vi "ResMgr-Request PriorityQueue.vi"(6 "Timeout In ms (5000 ms)":i32=5000, 7 "WatchDogQ":refnum<queue>, 8 "Error In":errorcluster caption="error in (no error)") -> (0 "error out":errorcluster, 3 "Priority Queue":T1)   [LabVIEW 2017, in "Communicable State Machine.lvlib"]
uses:
  Communicable State Machine.lvlib
  Priority Queue/Priority Queue.ctl
  Typedef/_Cross CSM State Data.ctl
  Typedef/_CSM_MSG_TYPE.ctl
  Typedef/_Cross CSM State Response.ctl
  Typedef/_CSM_Response Source Message.ctl
  Priority Queue/def-Data(LowPRI-Q).ctl
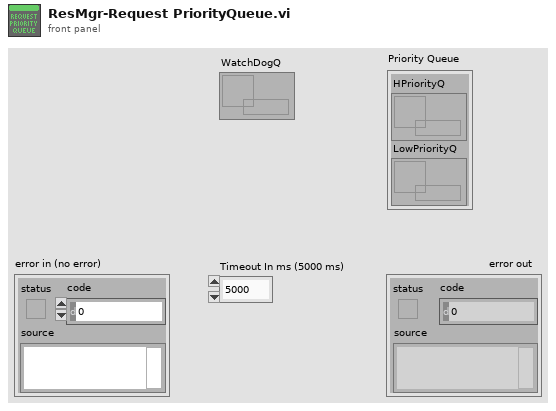
[diagram p1: front panel]
types:
  T1 = typedef "Communicable State Machine.lvlib/Priority Queue.ctl" = cluster{"HPriorityQ":refnum<queue>, "LowPriorityQ":refnum<queue>}
  T2 = cluster{"ResType":string, "RespQ":refnum<queue>, "Parameter":string, "WatchDogQ":refnum<queue>}
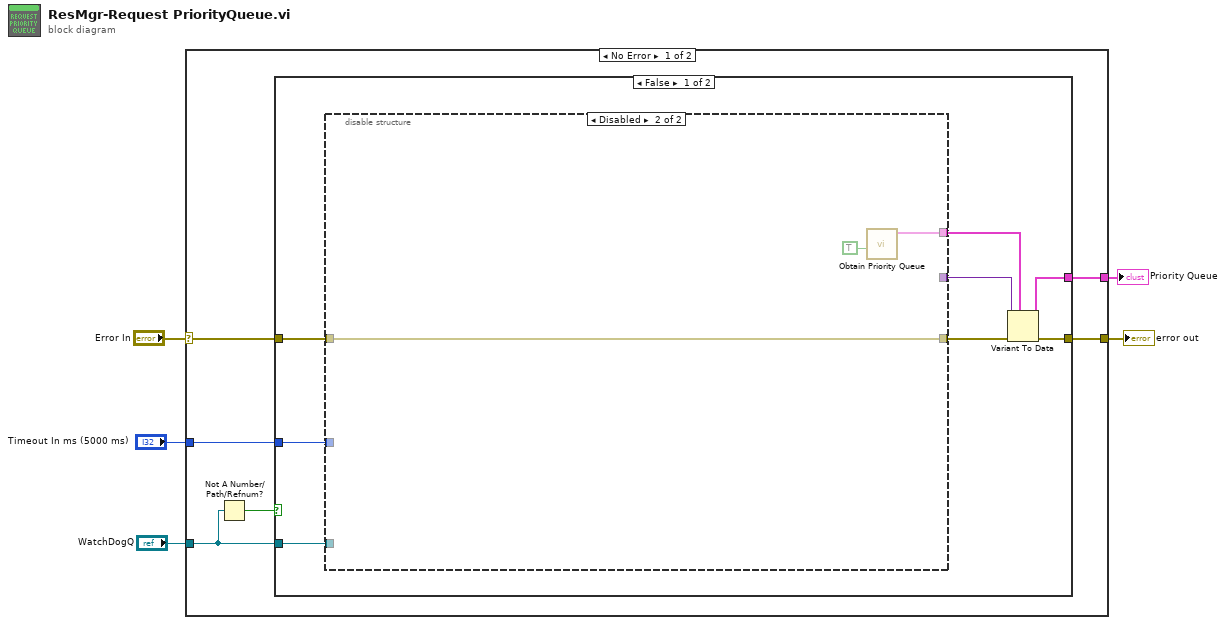
[diagram p0: block diagram]
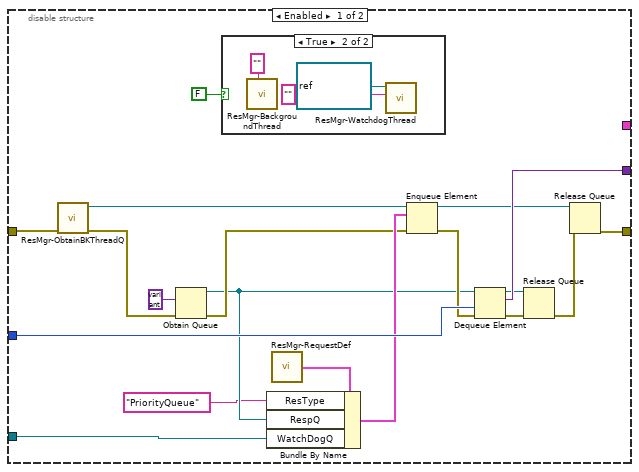
[diagram p2: hidden frame]
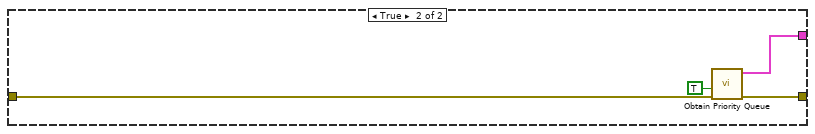
[diagram p4: hidden frame]
diagram:
  n1 = case shown="No Error" "Error In" {
    selector: "Error In" -> [w10 w49]
    tunnel: [w9 w49] -> w5
    tunnel: [w8 _] -> w1
    tunnel: "Timeout In ms (5000 ms)" -> [w11 _]
    tunnel: "WatchDogQ" -> [w7 _]
    frame No Error {
      n2 = Not A Number/Path/Refnum?(number/path/refnum=w7) -> (NaN/Path/Refnum?=w6:bool)
      n3 = case shown="False" w6 {
        tunnel: w11 -> [w18 _]
        tunnel: w10 -> [w17 w45]
        tunnel: w7 -> [w16 _]
        tunnel: [w15 w47] -> w9
        tunnel: [w12 w46] -> w8
        frame False {
          n4 = disable-structure shown="Disabled" {
            disable-tunnel: [w38 w44] -> w19
            disable-tunnel: w18 -> [w37 _]
            disable-tunnel: [w36 _] -> w14
            disable-tunnel: w17 -> [w23 w44]
            disable-tunnel: w16 -> [w22 _]
            disable-tunnel: [_ w42] -> w13
            frame Enabled {
              n5 = call "ResMgr-ObtainBKThreadQ.vi"("error in (no error)"=w23) -> ("error out"=w33:errorcluster, "ObtainBKThreadQ"=w34:refnum<queue>)  [unwired: 9 in]
              n6 = Obtain Queue(element data type=variant, error in (no error)=w33) -> (queue out=w24:refnum<queue>, error out=w32:errorcluster)  [unwired: 3 in, 1 out]
              n7 = case shown="True" FALSE {
                frame False {
                }
                frame True {
                  n8 = call "ResMgr-BackgroundThread.vi"("Name (Unnamed)"="" ("name (unnamed)")) -> ()  [unwired: 11 in]
                  n9 = call "ResMgr-WatchdogThread.vi"("From Who"="", "WatchDogQ"=refnum<queue> refnum) -> ()  [unwired: 10 in]
                }
              }
              n10 = call "ResMgr-RequestDef.vi"() -> ("ResMgr-RequestDef.ctl"=w20:T2)  [unwired: 2 in]
              n11 = Bundle By Name(cluster=w20, "ResType"="PriorityQueue", "RespQ"=w24, "WatchDogQ"=w22) -> (w35:T2)
              n12 = Enqueue Element(queue=w34, element=w35, error in (no error)=w32) -> (queue out=w28:refnum<queue>, error out=w31:errorcluster)  [unwired: 1 in, 1 out]
              n13 = Dequeue Element(queue=w24, timeout in ms (-1)=w37, error in (no error)=w31) -> (queue out=w29:refnum<queue>, element=w36:variant, error out=w30:errorcluster)  [unwired: 1 out]
              n14 = Release Queue(queue=w29, error in (no error)=w30) -> (error out=w27:errorcluster)  [unwired: 1 in, 2 out]
              n15 = Release Queue(queue=w28, error in (no error)=w27) -> (error out=w38:errorcluster)  [unwired: 1 in, 2 out]
            }
            frame Disabled {
              n16 = call "Obtain Priority Queue.vi"("Create If Not Found? (T)"=TRUE ("create if not found? (T)")) -> ("Priority Queue"=w42:T1)  [unwired: 8 in, 2 out]
            }
          }
          n17 = Variant To Data(error in=w19, type=w13, Variant=w14) -> (data=w12:T1, error out=w15:errorcluster)
        }
        frame True {
          n18 = call "Obtain Priority Queue.vi"("error in (no error)"=w45, "Create If Not Found? (T)"=TRUE ("create if not found? (T)")) -> ("error out"=w47:errorcluster, "Priority Queue"=w46:T1)  [unwired: 7 in, 1 out]
        }
      }
    }
    frame Error {
    }
  }
  "error out" <- w5
  "Priority Queue" <- w1
